vi "COMI AD Set Range.vi"(7 "vmax":sgl, 9 "vmin":sgl, 10 "ch":i32, 11 "hDevice":u32) -> (2 "function return":i32, 3 "hDevice out":u32)   [LabVIEW 2017, in "Comidll.lvlib"]
doc: "int (COMI_AD_SetRange) (HANDLE hDevice, int ch, float vmin, float vmax);"
uses:
  <userlib>/Comidll/Comidll.lvlib
  <userlib>/Comidll/Comidll.dll
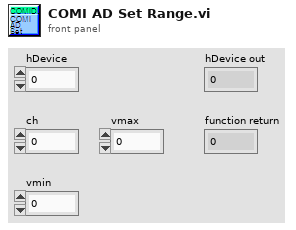
[diagram p1: front panel]
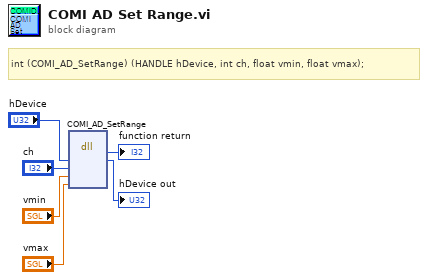
[diagram p0: block diagram]
diagram:
  # "int\t(COMI_AD_SetRange) (HANDLE hDevice, int ch, float vmin, float vmax);"
  n1 = dll-call lib="C:/Program Files/National Instruments/LabVIEW 2017/user.lib/Comidll/Comidll.*" fn="COMI_AD_SetRange"("hDevice"="hDevice", "ch"="ch", "vmin"="vmin", "vmax"="vmax") -> (→"function return":i32, "hDevice"=→"hDevice out":u32)  [unwired: 6 in, 2 out]
